vi "Create.vi"(7 "Direction":T1, 8 "error in (no error)":errorcluster, 9 "Custom Config Data":u8[](array[numeric]), 10 "Name":string, 11 "CIFTag in":refnum<class "CIF_NIChn_I64.lvclass">) -> (0 "error out":errorcluster, 3 "CIFTag out":refnum<class "CIF_NIChn_I64.lvclass">)   [LabVIEW 2021, in "CIF_NIChn_I64.lvclass"]
uses:
  CIF_NIChn_I64.lvclass
  D:/dev/CIF-LVCore/src/Channels/CIFChannels/CIFChannels.lvclass
  D:/dev/CIF-LVCore/src/Channels/CIF_NIChn/NIChn/CIF_NIChnl.lvclass
  CIFChannels/Typedef/Direction.ctl
  CIFChannels/Typedef/Disconnect Behavior.ctl
  CIFChannels/CIFChannels.lvclass/CIFChannels.ctl
  CIFChannels/Typedef/Channel State.ctl
  CIF_NIChn_I64.lvclass/CIF_NIChn_I64.ctl
  NIChn/CIF_NIChn.lvclass/CIF_NIChn.ctl
  02edcf3a-6131-4746-b933-e6a1af1fcb43.vi
  62a89f15-4a42-416c-81d4-6d85d5f7b5c9.vi
  85493118-15d5-4bf2-af7e-e73f555693b8.vi
  4a91887f-a40d-4172-85c4-b368c6e6f55f.vi
  CIFChannels/Accessors/Write Channel State.vi
  NIChn/Accessors/Write CIF Channel.vi
  CIFChannels/SubVIs/Get Type from Class.vi
  CIFChannels/Accessors/Write Type.vi
  CIFChannels/Accessors/Write Channel Class.vi
  CIFChannels/Accessors/Write Direction.vi
  CIFChannels/Accessors/Write Disconnect Behavior.vi
  CIFChannels/Accessors/Write Name.vi
  CIFChannels/Accessors/Write Custom Config Data.vi
  <vilib>/CIFChannels/SubVIs/Add Error.vi
  02edcf3a-6131-4746-b933-e6a1af1fcb43.vi/c28b0ead-42ad-4072-80a2-aca7f2bd7ce3.vi
  <vilib>/CIFChannels/SubVIs/CIFServices Fill In Error Info Ex.vi
  <vilib>/CIFChannels/SubVIs/Get dll Path.vi
  62a89f15-4a42-416c-81d4-6d85d5f7b5c9.vi/4bc1c15b-36ab-481f-b8dd-c64075ce723a.vi
  62a89f15-4a42-416c-81d4-6d85d5f7b5c9.vi/d83cb72b-7713-41fc-a3d1-682de79cf574.vi
  85493118-15d5-4bf2-af7e-e73f555693b8.vi/c28b0ead-42ad-4072-80a2-aca7f2bd7ce3.vi
  4a91887f-a40d-4172-85c4-b368c6e6f55f.vi/4bc1c15b-36ab-481f-b8dd-c64075ce723a.vi
  <vilib>/CIFChannels/SubVIs/Append Error Location.vi
  <vilib>/Utility/LVClass/Get LV Class Name.vi
  CIFChannels/CIFChannels.lvclass
  D:/dev/CIF-LVCore/src/Channels/CIF_NIChn/NIChn/CIF_NIChn.lvclass
  D:/dev/CIF-LVCore/src/Channels/CIF_NIChn/I64/CIF_NIChn_I64.lvclass
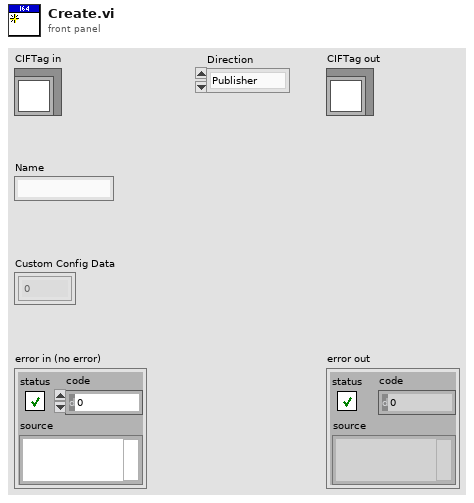
[diagram p1: front panel]
types:
  T1 = typedef "CIFChannels.lvclass/Direction.ctl" = enum16{"Publisher", "Subscriber"}
  T2 = typedef "CIFChannels.lvclass/Disconnect Behavior.ctl" = enum16{"Default value", "Last value", "Error with default"}
  T3 = typedef "CIFChannels.lvclass/Channel State.ctl" = enum16{"Creating", "Disconnected", "Connecting", "Connected", "Destroyed"}
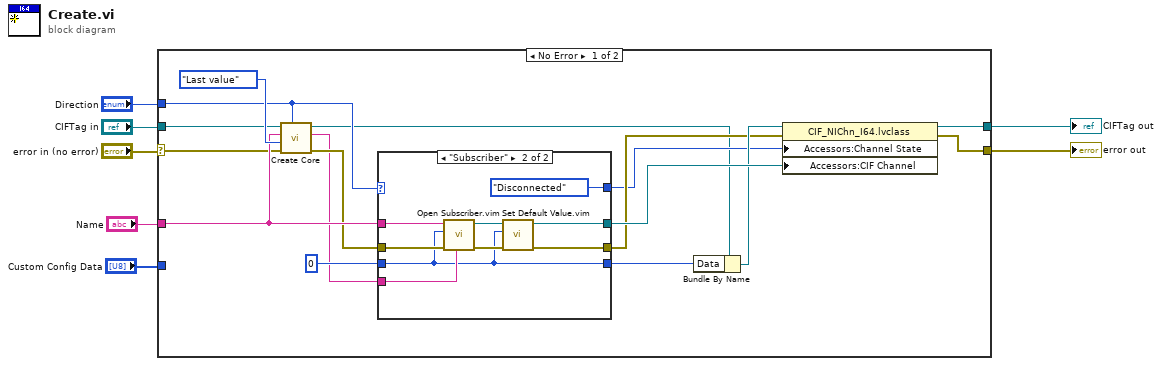
[diagram p0: block diagram]
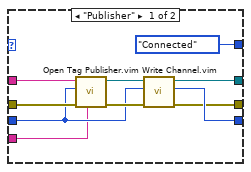
[diagram p2: hidden frame]
diagram:
  n1 = case shown="No Error" "error in (no error)" {
    selector: "error in (no error)" -> [w8 w44]
    tunnel: [w22 w44] -> w5
    tunnel: [w15 w43] -> w6
    tunnel: "CIFTag in" -> [w14 w43]
    tunnel: "Name" -> [w21 _]
    tunnel: "Direction" -> [w13 _]
    tunnel: "Custom Config Data" -> [_ _]
    frame No Error {
      n2 = call "Create Core.vi"("Direction"=w13, "error in (no error)"=w8, "Disconnect Behavior"=Disconnect_Behavior."Last value", "Name"=w21, "CIFChannels in"=w14) -> ("error out"=w20:errorcluster, "Channel Type"=w9:string, "CIFChannels out"=w11:refnum<class "CIF_NIChn_I64.lvclass">)  [unwired: 4 in]
      n3 = case shown="\"Subscriber\"" w13 {
        tunnel: w21 -> [w33 w41]
        tunnel: w20 -> [w32 w40]
        tunnel: [w29 w37] -> w19
        tunnel: i64 0 ("Default Value") -> [w28 w34]
        tunnel: [w27 w34] -> w17
        tunnel: [w26 w36] -> w16
        tunnel: w9 -> [w25 w35]
        tunnel: [Channel_State."Connected" ("Channel State") Channel_State."Disconnected" ("Channel State")] -> w12
        frame "Publisher" {
          n4 = call "Open Tag Publisher.vim"("Channel Type Description"=w25, "error in"=w32, "Input Type"=w28, "Channel Name"=w33) -> ("error out"=w30:errorcluster, "CIF Channel"=w31:refnum<k21>)  [unwired: 6 in]
          n5 = call "Write Channel.vim"("error in"=w30, "Data in"=w28, "CIF Channel in"=w31) -> ("error out"=w26:errorcluster, "Data out"=w27:i64, "CIF Channel out"=w29:refnum<k21>)  [unwired: 5 in, 1 out]
        }
        frame "Subscriber" {
          n6 = call "Open Subscriber.vim"("Channel Type Description"=w35, "error in"=w40, "Input Type"=w34, "Channel Name"=w41) -> ("error out"=w39:errorcluster, "CIF Channel"=w38:refnum<k21>)  [unwired: 6 in]
          n7 = call "Set Default Value.vim"("error in"=w39, "Data in"=w34, "CIF Channel in"=w38) -> ("error out"=w36:errorcluster, "CIF Channel out"=w37:refnum<k21>)  [unwired: 7 in]
        }
      }
      n8 = Bundle By Name(cluster=w11, "Data"=w17) -> (w18:refnum<class "CIF_NIChn_I64.lvclass">)
      n9 = property class="CIF_NIChn_I64.lvclass"(reference=w18, error in=w16, "Accessors:Channel State"=w12, "Accessors:CIF Channel"=w19) -> (reference out=w15:refnum<class "CIF_NIChn_I64.lvclass">, error out=w22:errorcluster)
    }
    frame Error {
    }
  }
  "error out" <- w5
  "CIFTag out" <- w6
